vi "adam-cmd-builder-2(SubVI).vi"(5 "Single/Multi Channel":bool, 7 "Channels":T2, 8 "Channel State Bit":bool, 9 "Channel Number in":i32 min=0 max=7 step=1, 10 "Device Address in":i32=1 min=0 max=100 step=2, 11 "Deliminator Char":string(combo)="#") -> (0 "Channel State String":string, 1 "Channel Number out":string, 2 "Device Address out":string, 3 "concatenated string":string, 4 "MultiCH-enable":T1(ring), 6 "SingleCH-enable":T1(ring)=enum."Disabled and Grayed Out")   [LabVIEW 2024]
panel:
  out "Channels As Number":u32
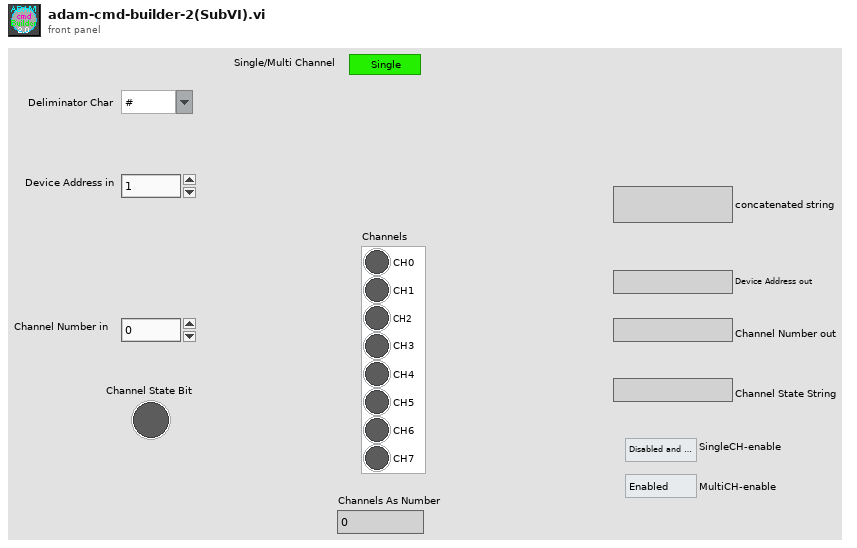
[diagram p1: front panel]
types:
  T1 = enum8{"Enabled", "Disabled", "Disabled and Grayed Out"}
  T2 = cluster{"CH0":bool, "CH1":bool, "CH2":bool, "CH3":bool, "CH4":bool, "CH5":bool, "CH6":bool, "CH7":bool}
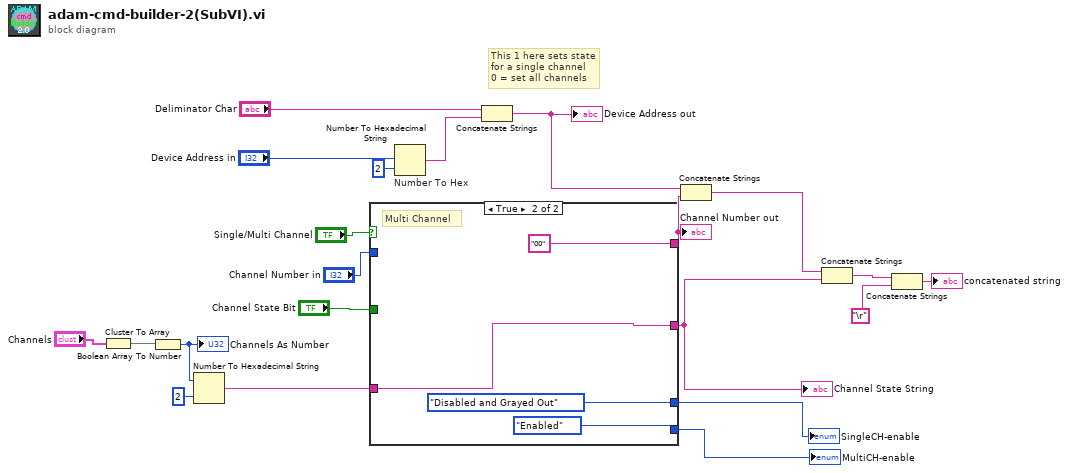
[diagram p0: block diagram]
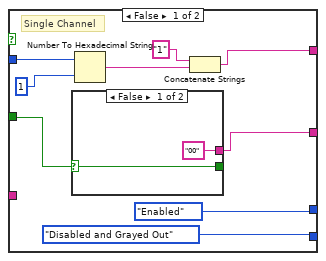
[diagram p2: hidden frame]
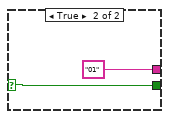
[diagram p3: hidden frame]
diagram:
  # "This 1 here sets state\nfor a single channel\n0 = set all channels"
  n1 = Cluster To Array(cluster="Channels") -> (array=w5:bool[])
  n2 = Boolean Array To Number(Boolean array=w5) -> (number=w6:u32)
  "Channels As Number" <- w6
  n3 = Number To Hexadecimal String(1:i16 2 ("width (-)"), 2:w6) -> (0:w3:string)
  n4 = case shown="True" "Single/Multi Channel" {
    tunnel: "Channel Number in" -> [w29 _]
    tunnel: [w26 "00"] -> w19
    tunnel: "Channel State Bit" -> [w24 _]
    tunnel: [w25 w37] -> w8
    tunnel: w3 -> [_ w37]
    tunnel: [T1."Enabled" ("Disabled") T1."Disabled and Grayed Out" ("Disabled")] -> w2
    tunnel: [T1."Disabled and Grayed Out" ("Disabled") T1."Enabled" ("Disabled")] -> w1
    frame False {
      # "Single Channel"
      n5 = case shown="False" w24 {
        selector: w24 -> [w31 w33]
        tunnel: ["00" "01"] -> w25
        tunnel: [w31 w33] -> _
        frame False {
        }
        frame True {
        }
      }
      n6 = Number To Hexadecimal String(1:i16 1 ("width (-)"), 2:w29) -> (0:w27:string)
      n7 = Concatenate Strings("1" ("string"), w27) -> (w26:string)
    }
    frame True {
      # "Multi Channel"
    }
  }
  "Channel State String" <- w8
  "Channel Number out" <- w19
  "SingleCH-enable" <- w2
  "MultiCH-enable" <- w1
  n8 = Number To Hexadecimal String "Number To Hex"(1:i16 2 ("width (-)"), 2:"Device Address in") -> (0:w15:string)
  n9 = Concatenate Strings("Deliminator Char", w15) -> (w12:string)
  "Device Address out" <- w12
  n10 = Concatenate Strings(w12, w19) -> (w20:string)
  n11 = Concatenate Strings(w20, w8) -> (w10:string)
  n12 = Concatenate Strings(w10, "\r") -> (→"concatenated string":string)
